vi "VI Tree.vi"   [LabVIEW 2020, in "eec 6700.lvlib"]
doc: "This instrument driver supports the Associated Power Technologies \"6000 Series Automated AC Power Source\".\n<B>Model Number</B> : 6705, 6710, 6720, 6630, 6640.\n\nThe VI Tree displays all the user-callable VIs of the instrument driver in an organized table."
uses:
  <instrlib>/eec 6700/eec 6700.lvlib
  <instrlib>/eec 6700/Public/Data/Read Test Data (Manual Mode).vi
  <instrlib>/eec 6700/Public/Data/Read (Timer).vi
panel:
  # "Please see diagram for eec 6700 Driver VI Tree"
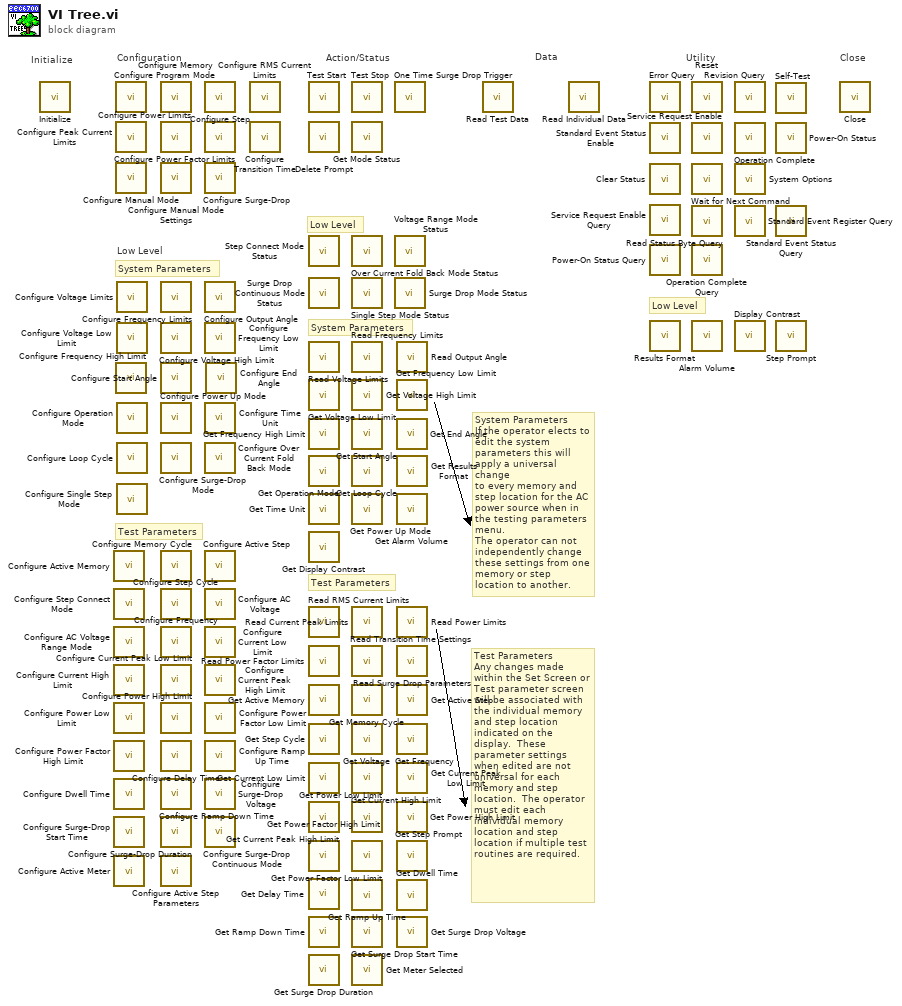
[diagram p0: block diagram]
diagram:
  # "Low Level"
  # "Low Level"
  # "Test Parameters\nAny changes made within the Set Screen or Test parameter screen will be associated with the individual memory and step location indicated on the display.  These parameter settings when edited are not universal for each memory and step location.  The operator must edit each individual memory location and step location if multiple test routines are required."
  # "System Parameters\nIf the operator elects to edit the system parameters this will apply a universal change \nto every memory and step location for the AC power source when in the testing parameters\nmenu.\nThe operator can not independently change these settings from one memory or step location to another."
  # "Test Parameters"
  # "System Parameters"
  # "System Parameters"
  # "Test Parameters"
  # "Low Level"
  # "Configuration"
  # "Utility"
  # "Data"
  # "Action/Status"
  # "Close"
  # "Initialize"
  n1 = call <instrlib>:"Initialize.vi"() -> ()  [unwired: 14 in, 2 out]
  n2 = call <instrlib>:"Configure Active Memory.vi"() -> ()  [unwired: 14 in, 2 out]
  n3 = call <instrlib>:"Configure Step Connect Mode.vi"() -> ()  [unwired: 14 in, 2 out]
  n4 = call <instrlib>:"Configure AC Voltage Range Mode.vi"() -> ()  [unwired: 14 in, 2 out]
  n5 = call <instrlib>:"Configure Current High Limit.vi"() -> ()  [unwired: 14 in, 2 out]
  n6 = call <instrlib>:"Configure Power Low Limit.vi"() -> ()  [unwired: 14 in, 2 out]
  n7 = call <instrlib>:"Configure Power Factor High Limit.vi"() -> ()  [unwired: 14 in, 2 out]
  n8 = call <instrlib>:"Configure Dwell Time.vi"() -> ()  [unwired: 14 in, 2 out]
  n9 = call <instrlib>:"Configure Surge-Drop Start Time.vi"() -> ()  [unwired: 14 in, 2 out]
  n10 = call <instrlib>:"Configure Active Meter.vi"() -> ()  [unwired: 14 in, 2 out]
  n11 = call <instrlib>:"Configure Program Mode.vi"() -> ()  [unwired: 14 in, 2 out]
  n12 = call <instrlib>:"Configure Peak Current Limits.vi"() -> ()  [unwired: 14 in, 2 out]
  n13 = call <instrlib>:"Configure Manual Mode.vi"() -> ()  [unwired: 14 in, 2 out]
  n14 = call <instrlib>:"Configure Frequency High Limit.vi"() -> ()  [unwired: 14 in, 2 out]
  n15 = call <instrlib>:"Configure Voltage Limits.vi"() -> ()  [unwired: 14 in, 2 out]
  n16 = call <instrlib>:"Configure Voltage Low Limit.vi"() -> ()  [unwired: 14 in, 2 out]
  n17 = call <instrlib>:"Configure Operation Mode.vi"() -> ()  [unwired: 14 in, 2 out]
  n18 = call <instrlib>:"Configure Loop Cycle.vi"() -> ()  [unwired: 14 in, 2 out]
  n19 = call <instrlib>:"Configure Single Step Mode.vi"() -> ()  [unwired: 14 in, 2 out]
  n20 = call <instrlib>:"Configure Memory.vi"() -> ()  [unwired: 14 in, 2 out]
  n21 = call <instrlib>:"Configure Power Limits.vi"() -> ()  [unwired: 14 in, 2 out]
  n22 = call <instrlib>:"Configure Manual Mode Settings.vi"() -> ()  [unwired: 14 in, 2 out]
  n23 = call <instrlib>:"Configure Frequency Limits.vi"() -> ()  [unwired: 14 in, 2 out]
  n24 = call <instrlib>:"Configure Voltage High Limit.vi"() -> ()  [unwired: 14 in, 2 out]
  n25 = call <instrlib>:"Configure Start Angle.vi"() -> ()  [unwired: 14 in, 2 out]
  n26 = call <instrlib>:"Configure Power Up Mode.vi"() -> ()  [unwired: 14 in, 2 out]
  n27 = call <instrlib>:"Configure Surge-Drop Mode.vi"() -> ()  [unwired: 14 in, 2 out]
  n28 = call <instrlib>:"Configure Memory Cycle.vi"() -> ()  [unwired: 14 in, 2 out]
  n29 = call <instrlib>:"Configure Step Cycle.vi"() -> ()  [unwired: 14 in, 2 out]
  n30 = call <instrlib>:"Configure Frequency.vi"() -> ()  [unwired: 14 in, 2 out]
  n31 = call <instrlib>:"Configure Current Peak Low Limit.vi"() -> ()  [unwired: 14 in, 2 out]
  n32 = call <instrlib>:"Configure Power High Limit.vi"() -> ()  [unwired: 14 in, 2 out]
  n33 = call <instrlib>:"Configure Delay Time.vi"() -> ()  [unwired: 14 in, 2 out]
  n34 = call <instrlib>:"Configure Ramp Down Time.vi"() -> ()  [unwired: 14 in, 2 out]
  n35 = call <instrlib>:"Configure Surge-Drop Duration.vi"() -> ()  [unwired: 14 in, 2 out]
  n36 = call <instrlib>:"Configure Active Step Parameters.vi"() -> ()  [unwired: 14 in, 2 out]
  n37 = call <instrlib>:"Configure Step.vi"() -> ()  [unwired: 14 in, 2 out]
  n38 = call <instrlib>:"Configure Power Factor Limits.vi"() -> ()  [unwired: 14 in, 2 out]
  n39 = call <instrlib>:"Configure Surge-Drop.vi"() -> ()  [unwired: 14 in, 2 out]
  n40 = call <instrlib>:"Configure Output Angle.vi"() -> ()  [unwired: 14 in, 2 out]
  n41 = call <instrlib>:"Configure Frequency Low Limit.vi"() -> ()  [unwired: 14 in, 2 out]
  n42 = call <instrlib>:"Configure Time Unit.vi"() -> ()  [unwired: 14 in, 2 out]
  n43 = call <instrlib>:"Configure Over Current Fold Back Mode.vi"() -> ()  [unwired: 14 in, 2 out]
  n44 = call <instrlib>:"Configure Active Step.vi"() -> ()  [unwired: 14 in, 2 out]
  n45 = call <instrlib>:"Configure AC Voltage.vi"() -> ()  [unwired: 14 in, 2 out]
  n46 = call <instrlib>:"Configure Current Low Limit.vi"() -> ()  [unwired: 14 in, 2 out]
  n47 = call <instrlib>:"Configure Current Peak High Limit.vi"() -> ()  [unwired: 14 in, 2 out]
  n48 = call <instrlib>:"Configure Power Factor Low Limit.vi"() -> ()  [unwired: 14 in, 2 out]
  n49 = call <instrlib>:"Configure Ramp Up Time.vi"() -> ()  [unwired: 14 in, 2 out]
  n50 = call <instrlib>:"Configure Surge-Drop Voltage.vi"() -> ()  [unwired: 14 in, 2 out]
  n51 = call <instrlib>:"Configure Surge-Drop Continuous Mode.vi"() -> ()  [unwired: 14 in, 2 out]
  n52 = call <instrlib>:"Configure End Angle.vi"() -> ()  [unwired: 14 in, 2 out]
  n53 = call <instrlib>:"Configure RMS Current Limits.vi"() -> ()  [unwired: 14 in, 2 out]
  n54 = call <instrlib>:"Configure Transition Time.vi"() -> ()  [unwired: 14 in, 2 out]
  n55 = call <instrlib>:"Test Start.vi"() -> ()  [unwired: 14 in, 2 out]
  n56 = call <instrlib>:"Delete Prompt.vi"() -> ()  [unwired: 14 in, 2 out]
  n57 = call <instrlib>:"Step Connect Mode Status.vi"() -> ()  [unwired: 13 in, 3 out]
  n58 = call <instrlib>:"Surge Drop Continuous Mode Status.vi"() -> ()  [unwired: 13 in, 3 out]
  n59 = call <instrlib>:"Read Voltage Limits.vi"() -> ()  [unwired: 12 in, 4 out]
  n60 = call <instrlib>:"Get Voltage Low Limit.vi"() -> ()  [unwired: 13 in, 3 out]
  n61 = call <instrlib>:"Get Frequency High Limit.vi"() -> ()  [unwired: 13 in, 3 out]
  n62 = call <instrlib>:"Get Operation Mode.vi"() -> ()  [unwired: 13 in, 3 out]
  n63 = call <instrlib>:"Get Time Unit.vi"() -> ()  [unwired: 13 in, 3 out]
  n64 = call <instrlib>:"Get Display Contrast.vi"() -> ()  [unwired: 13 in, 3 out]
  n65 = call <instrlib>:"Read RMS Current Limits.vi"() -> ()  [unwired: 12 in, 4 out]
  n66 = call <instrlib>:"Read Power Factor Limits.vi"() -> ()  [unwired: 12 in, 4 out]
  n67 = call <instrlib>:"Get Active Memory.vi"() -> ()  [unwired: 13 in, 3 out]
  n68 = call <instrlib>:"Get Step Cycle.vi"() -> ()  [unwired: 13 in, 3 out]
  n69 = call <instrlib>:"Get Current Low Limit.vi"() -> ()  [unwired: 13 in, 3 out]
  n70 = call <instrlib>:"Get Current Peak High Limit.vi"() -> ()  [unwired: 13 in, 3 out]
  n71 = call <instrlib>:"Get Power Factor High Limit.vi"() -> ()  [unwired: 13 in, 3 out]
  n72 = call <instrlib>:"Get Delay Time.vi"() -> ()  [unwired: 13 in, 3 out]
  n73 = call <instrlib>:"Get Ramp Down Time.vi"() -> ()  [unwired: 13 in, 3 out]
  n74 = call <instrlib>:"Get Surge Drop Duration.vi"() -> ()  [unwired: 13 in, 3 out]
  n75 = call <instrlib>:"Test Stop.vi"() -> ()  [unwired: 14 in, 2 out]
  n76 = call <instrlib>:"Get Mode Status.vi"() -> ()  [unwired: 8 in, 8 out]
  n77 = call <instrlib>:"Over Current Fold Back Mode Status.vi"() -> ()  [unwired: 13 in, 3 out]
  n78 = call <instrlib>:"Single Step Mode Status.vi"() -> ()  [unwired: 13 in, 3 out]
  n79 = call <instrlib>:"Read Frequency Limits.vi"() -> ()  [unwired: 12 in, 4 out]
  n80 = call <instrlib>:"Get Voltage High Limit.vi"() -> ()  [unwired: 13 in, 3 out]
  n81 = call <instrlib>:"Get Start Angle.vi"() -> ()  [unwired: 13 in, 3 out]
  n82 = call <instrlib>:"Get Loop Cycle.vi"() -> ()  [unwired: 13 in, 3 out]
  n83 = call <instrlib>:"Get Power Up Mode.vi"() -> ()  [unwired: 13 in, 3 out]
  n84 = call <instrlib>:"Read Current Peak Limits.vi"() -> ()  [unwired: 12 in, 4 out]
  n85 = call <instrlib>:"Read Transition Time Settings.vi"() -> ()  [unwired: 10 in, 6 out]
  n86 = call <instrlib>:"Get Memory Cycle.vi"() -> ()  [unwired: 13 in, 3 out]
  n87 = call <instrlib>:"Get Voltage.vi"() -> ()  [unwired: 13 in, 3 out]
  n88 = call <instrlib>:"Get Current High Limit.vi"() -> ()  [unwired: 13 in, 3 out]
  n89 = call <instrlib>:"Get Power Low Limit.vi"() -> ()  [unwired: 13 in, 3 out]
  n90 = call <instrlib>:"Get Power Factor Low Limit.vi"() -> ()  [unwired: 13 in, 3 out]
  n91 = call <instrlib>:"Get Ramp Up Time.vi"() -> ()  [unwired: 13 in, 3 out]
  n92 = call <instrlib>:"Get Surge Drop Start Time.vi"() -> ()  [unwired: 13 in, 3 out]
  n93 = call <instrlib>:"Get Meter Selected.vi"() -> ()  [unwired: 13 in, 3 out]
  n94 = call <instrlib>:"One Time Surge Drop Trigger.vi"() -> ()  [unwired: 14 in, 2 out]
  n95 = call <instrlib>:"Voltage Range Mode Status.vi"() -> ()  [unwired: 13 in, 3 out]
  n96 = call <instrlib>:"Surge Drop Mode Status.vi"() -> ()  [unwired: 13 in, 3 out]
  n97 = call <instrlib>:"Read Output Angle.vi"() -> ()  [unwired: 12 in, 4 out]
  n98 = call <instrlib>:"Get Frequency Low Limit.vi"() -> ()  [unwired: 13 in, 3 out]
  n99 = call <instrlib>:"Get End Angle.vi"() -> ()  [unwired: 13 in, 3 out]
  n100 = call <instrlib>:"Get Results Format.vi"() -> ()  [unwired: 13 in, 3 out]
  n101 = call <instrlib>:"Get Alarm Volume.vi"() -> ()  [unwired: 13 in, 3 out]
  n102 = call <instrlib>:"Read Power Limits.vi"() -> ()  [unwired: 12 in, 4 out]
  n103 = call <instrlib>:"Read Surge Drop Parameters.vi"() -> ()  [unwired: 11 in, 5 out]
  n104 = call <instrlib>:"Get Active Step.vi"() -> ()  [unwired: 13 in, 3 out]
  n105 = call <instrlib>:"Get Frequency.vi"() -> ()  [unwired: 13 in, 3 out]
  n106 = call <instrlib>:"Get Current Peak Low Limit.vi"() -> ()  [unwired: 13 in, 3 out]
  n107 = call <instrlib>:"Get Power High Limit.vi"() -> ()  [unwired: 13 in, 3 out]
  n108 = call <instrlib>:"Get Step Prompt.vi"() -> ()  [unwired: 13 in, 3 out]
  n109 = call <instrlib>:"Get Dwell Time.vi"() -> ()  [unwired: 13 in, 3 out]
  n110 = call <instrlib>:"Get Surge Drop Voltage.vi"() -> ()  [unwired: 13 in, 3 out]
  n111 = call-poly <instrlib>:"Read Test Data.vi"() -> ()  [unwired: 13 in, 3 out]
  n112 = call-poly <instrlib>:"Read Individual Data.vi"() -> ()  [unwired: 13 in, 3 out]
  n113 = call <instrlib>:"Error Query.vi"() -> ()  [unwired: 12 in, 4 out]
  n114 = call <instrlib>:"Standard Event Status Enable.vi"() -> ()  [unwired: 14 in, 2 out]
  n115 = call <instrlib>:"Clear Status.vi"() -> ()  [unwired: 14 in, 2 out]
  n116 = call <instrlib>:"Service Request Enable Query.vi"() -> ()  [unwired: 13 in, 3 out]
  n117 = call <instrlib>:"Power-On Status Query.vi"() -> ()  [unwired: 13 in, 3 out]
  n118 = call <instrlib>:"Results Format.vi"() -> ()  [unwired: 14 in, 2 out]
  n119 = call <instrlib>:"Reset.vi"() -> ()  [unwired: 14 in, 2 out]
  n120 = call <instrlib>:"Service Request Enable.vi"() -> ()  [unwired: 14 in, 2 out]
  n121 = call <instrlib>:"Wait for Next Command.vi"() -> ()  [unwired: 14 in, 2 out]
  n122 = call <instrlib>:"Read Status Byte Query.vi"() -> ()  [unwired: 13 in, 3 out]
  n123 = call <instrlib>:"Operation Complete Query.vi"() -> ()  [unwired: 13 in, 3 out]
  n124 = call <instrlib>:"Alarm Volume.vi"() -> ()  [unwired: 14 in, 2 out]
  n125 = call <instrlib>:"Revision Query.vi"() -> ()  [unwired: 11 in, 5 out]
  n126 = call <instrlib>:"Operation Complete.vi"() -> ()  [unwired: 14 in, 2 out]
  n127 = call <instrlib>:"System Options.vi"() -> ()  [unwired: 10 in, 2 out]
  n128 = call <instrlib>:"Standard Event Register Query.vi"() -> ()  [unwired: 13 in, 3 out]
  n129 = call <instrlib>:"Display Contrast.vi"() -> ()  [unwired: 14 in, 2 out]
  n130 = call <instrlib>:"Self-Test.vi"() -> ()  [unwired: 12 in, 4 out]
  n131 = call <instrlib>:"Power-On Status.vi"() -> ()  [unwired: 14 in, 2 out]
  n132 = call <instrlib>:"Standard Event Status Query.vi"() -> ()  [unwired: 13 in, 3 out]
  n133 = call <instrlib>:"Step Prompt.vi"() -> ()  [unwired: 14 in, 2 out]
  n134 = call <instrlib>:"Close.vi"() -> ()  [unwired: 15 in, 1 out]
